vi "Get Width.vi"(8 "error in (no error)":errorcluster, 11 "TermBuffer in":refnum<class "TermBuffer.lvclass">) -> (0 "error out":errorcluster, 2 "Width":i32, 3 "TermBuffer out":refnum<class "TermBuffer.lvclass">)   [LabVIEW 2020, in "Terminal.lvlib" / "TermBuffer.lvclass"]
doc: "Returns the column count for scren buffers and always returns 0 for scrollback buffers since lines can have variable lengths."
uses:
  TermBuffer.lvclass
  TermBuffer.lvclass/TermBuffer.ctl
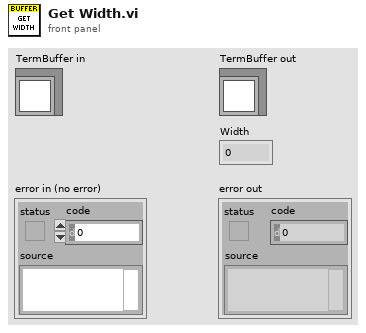
[diagram p1: front panel]
types:
  T1 = typedef "Terminal.lvlib/TermBuffer.lvclass/Ref Data.ctl" = cluster{"Lines":refnum<class "TermLine.lvclass">[], "Rows":i32, "Cols":i32}
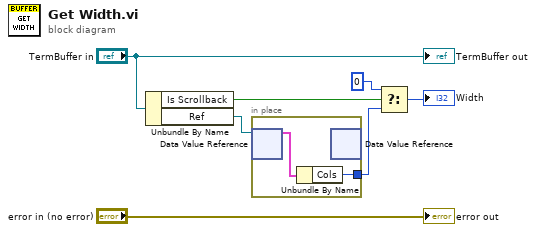
[diagram p0: block diagram]
diagram:
  n1 = Unbundle By Name("TermBuffer in") -> ("Is Scrollback"=w4:bool, "Ref"=w6:refnum<data-value>)
  n2 = in-place {
    in-place-border: [w8] -> w3
    n3 = in-place-dvr #1(w6) -> (w9:T1)  [unwired: 1 out]
    n4 = Unbundle By Name(w9) -> ("Cols"=w8:i32)
    n5 = in-place-dvr #1() -> ()  [unwired: 1 in, 2 out]
  }
  n6 = Select(t=0, s=w4, f=w3) -> (s? t:f=→"Width":i32)
  "error out" <- "error in (no error)"
  "TermBuffer out" <- "TermBuffer in"
